vi "conv.csv.to.ob.cmd.vi"(11 "String":string="Type, Side, OrderId, Quantity, Symbol, Price, ExeQty, CancelQty, RemQty, Seconds, Nanoseconds, Add, Edit, Remove\nAddOrder, Buy, 0x31, 100, AAPL, 100.20, 0, 0, 0, 0, 0, True, False, False\nAddOrder, Buy, 0x32, 200, AAPL, 100.25, 0, 0, 0, 0, 0, True, False, False\nAddOrder, Buy, 0x33, 25, AAPL, 100.23, 0, 0, 0, 0, 0, True, False, False") -> (3 "OrderBook.Commands.out":T1[](array[typedef])=[{"type"=enum."AddOrder", "side"=102, "orderId "=49, "quantity"=100, "symbol"=4702127773838221344, "price"=1002000, "executed.qty"=0, "canceled.qty"=0, "remaining.qty"=0, "seconds"=0, "nanoseconds"=0, "Add"=TRUE, "Edit"=FALSE, "Remove"=FALSE, "seq no"=0}, {"type"=enum."AddOrder", "side"=102, "orderId "=50, "quantity"=200, "symbol"=4702127773838221344, "price"=1002500, "executed.qty"=0, "canceled.qty"=0, "remaining.qty"=0, "seconds"=0, "nanoseconds"=0, "Add"=TRUE, "Edit"=FALSE, "Remove"=FALSE, "seq no"=0}, {"type"=enum."AddOrder", "side"=102, "orderId "=51, "quantity"=25, "symbol"=4702127773838221344, "price"=1002300, "executed.qty"=0, "canceled.qty"=0, "remaining.qty"=0, "seconds"=0, "nanoseconds"=0, "Add"=TRUE, "Edit"=FALSE, "Remove"=TRUE, "seq no"=0}] {"symbol" format="%.0x"; "orderId" format="%.0x"; "side" format="%.0x"})   [LabVIEW 2020, in "fpganow.common.host.lvlib"]
uses:
  fpganow.common.host.lvlib
  fpga/orderbook.command.ctl
  fpga/orderbook.command.type.ctl
  fpga/fpganow.common.fpga.lvlib
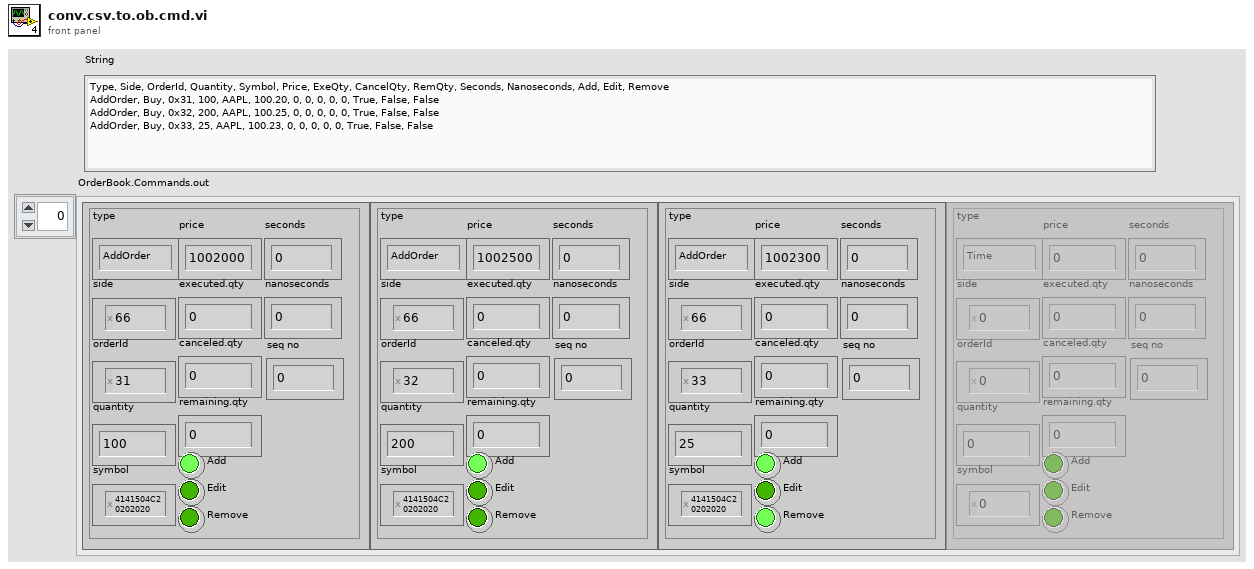
[diagram p1: front panel]
types:
  T1 = typedef "fpganow.common.fpga.lvlib/orderbook.command.ctl" = cluster{"type":T2, "side":u8, "orderId ":u64, "quantity":u32, "symbol":u64, "price":u64, "executed.qty":u32, "canceled.qty":u32, "remaining.qty":u32, "seconds":u64, "nanoseconds":u64, "Add":bool, "Edit":bool, "Remove":bool, "seq no":u32}
  T2 = typedef "fpganow.common.fpga.lvlib/orderbook.command.type.ctl" = enum8{"Time", "AddOrder", "OrderExecuted", "OrderExecutedAtPrice", "ReduceSize", "ModifyOrder", "DeleteOrder", "Get.Everything", "Get.All.Orders", "Get.Top"}
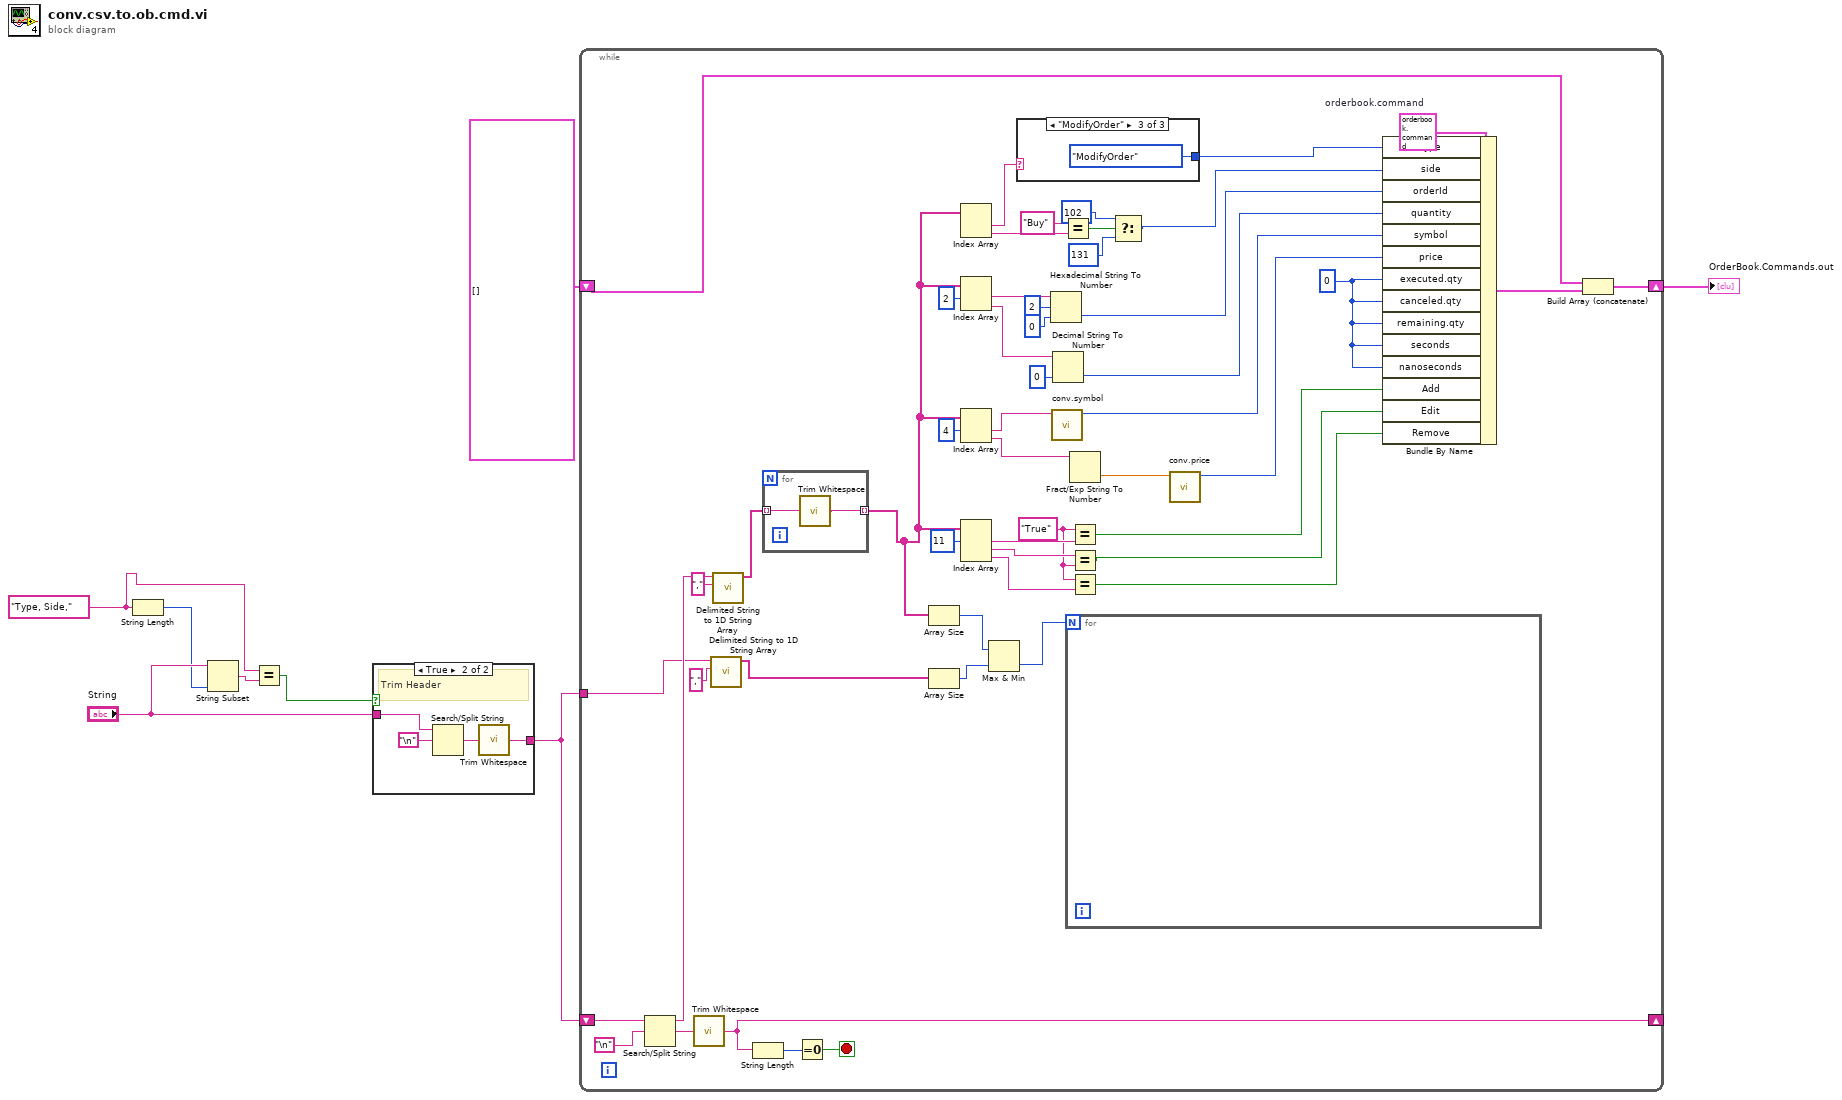
[diagram p0: block diagram]
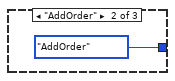
[diagram p4: hidden frame]
diagram:
  w1 = "Type, Side,"
  n1 = String Length(string=w1) -> (length=w4:i32)
  n2 = String Subset(string="String", length (rest)=w4) -> (substring=w3:string)  [unwired: 1 in]
  n3 = Equal?(x=w1, y=w3) -> (x = y?=w2:bool)
  n4 = case shown="True" w2 {
    tunnel: [w9 w11] -> w6
    tunnel: "String" -> [w9 w10]
    frame False {
      # "No Header"
    }
    frame True {
      # "Trim Header"
      n5 = Search/Split String(string=w10, search string/char (-)="\n") -> (match + rest of string=w12:string)  [unwired: 1 in, 2 out]
      n6 = call <vilib>:"Trim Whitespace.vi"("string"=w12) -> ("trimmed string"=w11:string)  [unwired: 1 in]
    }
  }
  n7 = while {
    shift-right: [w61] -> _
    shift-left: w6 -> [w64]
    shift-right: [w22] -> w8
    shift-left: T1[] [] -> [w21]
    tunnel: w6 -> [w18]
    stop <- w59 stop-if-true
    w26 = "True" ("x")
    w23 = u32 0 ("executed.qty")
    w55 = T1 {"type"=enum."Time", "side"=0, "orderId "=0, "quantity"=0, "symbol"=0, "price"=0, "executed.qty"=0, "canceled.qty"=0, "remaining.qty"=0, "seconds"=0, "nanoseconds"=0, "Add"=FALSE, "Edit"=FALSE, "Remove"=FALSE, "seq no"=0}  # orderbook.command
    n8 = Search/Split String(string=w64, search string/char (-)="\n") -> (substring before match=w58:string, match + rest of string=w62:string)  [unwired: 1 in, 1 out]
    n9 = call <vilib>:"Trim Whitespace.vi"("string"=w62) -> ("trimmed string"=w61:string)  [unwired: 1 in]
    n10 = call <vilib>:"Delimited String to 1D String Array.vi"("delimiter"=",", "delimited string"=w18) -> ("string array"=w17:string[])  [unwired: 9 in]
    n11 = call <vilib>:"Delimited String to 1D String Array.vi"("delimiter"=",", "delimited string"=w58) -> ("string array"=w43:string[])  [unwired: 9 in]
    n12 = String Length(string=w61) -> (length=w60:i32)
    n13 = for {
      tunnel: w43 -> [w66] mode=indexing
      tunnel: [w65] -> w20 mode=indexing
      n14 = call <vilib>:"Trim Whitespace.vi"("string"=w66) -> ("trimmed string"=w65:string)  [unwired: 1 in]
    }
    n15 = Equal To 0?(x=w60) -> (x = 0?=w59:bool)
    n16 = Array Size(array=w20) -> (size(s)=w16:i32)
    n17 = Array Size(array=w17) -> (size(s)=w15:i32)
    n18 = Index Array(array=w20) -> (element #1=w56:string, element #2=w53:string)  [unwired: 2 in]
    n19 = Index Array(array=w20, index #1=2 ("index")) -> (element #1=w46:string, element #2=w41:string)  [unwired: 1 in]
    n20 = Index Array(array=w20, index #1=4 ("index")) -> (element #1=w38:string, element #2=w35:string)  [unwired: 1 in]
    n21 = Index Array(array=w20, index #1=11 ("index")) -> (element #1=w30:string, element #2=w28:string, element #3=w27:string)  [unwired: 2 in]
    n22 = Max & Min(x=w16, y=w15) -> (min(x,y)=w14:i32)  [unwired: 1 out]
    n23 = case shown="\"ModifyOrder\"" w56 {
      tunnel: [_ orderbook.command.type."AddOrder" ("type") orderbook.command.type."ModifyOrder" ("type")] -> w54
      frame "False", Default {
      }
      frame "AddOrder" {
      }
      frame "ModifyOrder" {
      }
    }
    n24 = Hexadecimal String To Number(string=w46, offset=2, default (0uL)=u64 0 ("default (0 U32)")) -> (number=w44:u64)  [unwired: 1 out]
    n25 = call "conv.symbol.vi"("symbol.in"=w38) -> ("symbol.out"=w37:u64)  [unwired: 10 in]
    n26 = Decimal String To Number(string=w41, default (0L)=u32 0 ("default (0 I32)")) -> (number=w39:u32)  [unwired: 1 in, 1 out]
    n27 = Equal?(x="Buy", y=w53) -> (x = y?=w51:bool)
    n28 = for {
      N: w14 -> [_]
    }
    n29 = Fract/Exp String To Number(string=w35) -> (number=w34:dbl)  [unwired: 3 in, 1 out]
    n30 = Equal?(x=w26, y=w30) -> (x = y?=w29:bool)
    n31 = Equal?(x=w28, y=w26) -> (x = y?=w25:bool)
    n32 = Equal?(x=w26, y=w27) -> (x = y?=w24:bool)
    n33 = Select(t=u8 102 ("side"), s=w51, f=u8 131 ("side")) -> (s? t:f=w48:u8)
    n34 = call "conv.price.vi"("price.in"=w34) -> ("price.out"=w36:u64)  [unwired: 10 in]
    n35 = Bundle By Name(cluster=w55, "type"=w54, "side"=w48, "orderId"=w44, "quantity"=w39, "symbol"=w37, "price"=w36, "executed.qty"=w23, "canceled.qty"=w23, "remaining.qty"=w23, "seconds"=w23, "nanoseconds"=w23, "Add"=w29, "Edit"=w25, "Remove"=w24) -> (w31:T1)
    n36 = Build Array (concatenate)(w21, w31) -> (w22:T1[])
  }
  "OrderBook.Commands.out" <- w8
